vi "GetInputShapeDimCount.vi"(8 "error in (no error)":errorcluster, 10 "inputIndex":i32, 11 "session id in":i32) -> (0 "error out":errorcluster, 2 "InputShapeDimCount":i32, 3 "session id out":i32)   [LabVIEW 2017, in "libonnx_wrapper.lvlib"]
doc: "/**\n * @brief Получить количество размерностей входного тензора\n * \n * Возвращает ранг тензора (число измерений). Например:\n * - Вектор [10] имеет 1 размерность\n * - Матрица [1, 10] имеет 2 размерности\n * - Изображение [1, 3, 224, 224] имеет 4 размерности\n * \n * @param sessionId [IN] ID сессии\n * @param inputIndex [IN] Индекс входа (0-based)\n * \n * @return int32: Количество размерностей (1, 2, 3, 4, ...)\n * @return int32: 0 если сессия не найдена или индекс неверен\n */\nint GetInputShapeDimCount(int sessionId, int inputIndex);"
uses:
  libonnx_wrapper.lvlib
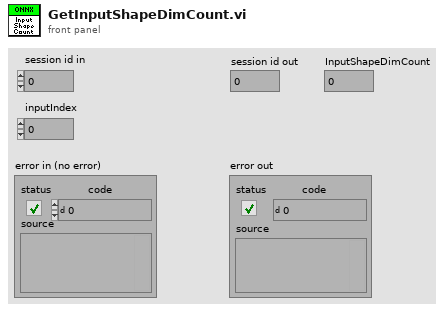
[diagram p1: front panel]
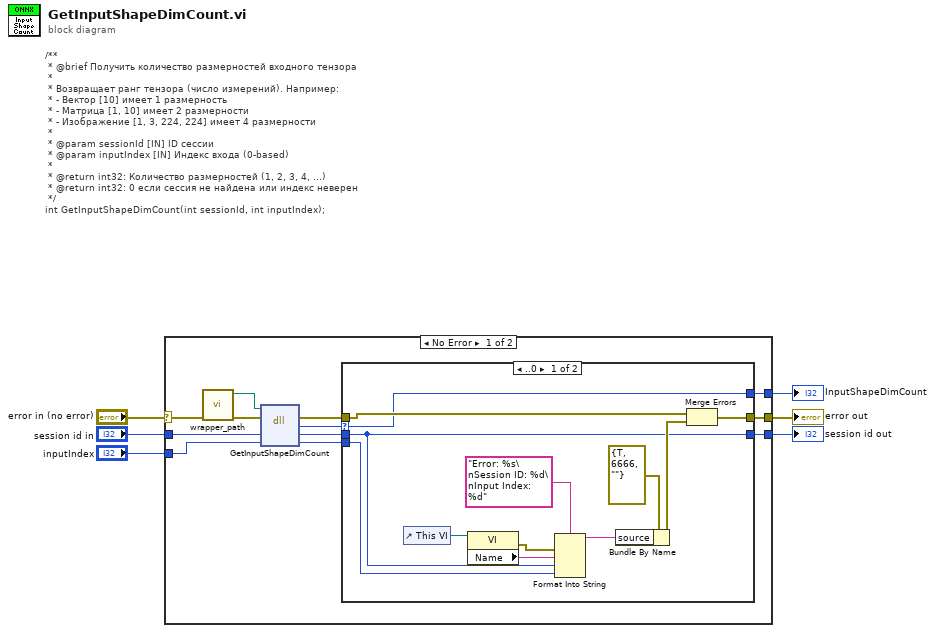
[diagram p0: block diagram]
diagram:
  # "/**\n * @brief Получить количество размерностей входного тензора\n * \n * Возвращает ранг тензора (число измерений). Например:\n * - Вектор [10] имеет 1 размерность\n * - Матрица [1, 10] имеет 2 размерности\n * - Изображение [1, 3, 224, 224] имеет 4 размерности\n * \n * @param sessionId [IN] ID сессии\n * @param inputIndex [IN] Индекс входа (0-based)\n * \n * @return int32: Количество размерностей (1, 2, 3, 4, ...)\n * @return int32: 0 если сессия не найдена или индекс неверен\n */\nint GetInputShapeDimCount(int sessionId, int inputIndex);"
  n1 = case shown="No Error" "error in (no error)" {
    selector: "error in (no error)" -> [w7 w35]
    tunnel: "inputIndex" -> [w18 _]
    tunnel: "session id in" -> [w16 w34]
    tunnel: [w13 w35] -> w4
    tunnel: [w9 _] -> w3
    tunnel: [w8 w34] -> w2
    frame No Error {
      n2 = call "wrapper_path.vi"("error in (no error)"=w7) -> ("error out"=w15:errorcluster, "wrapper path"=w17:path)  [unwired: 9 in]
      n3 = dll-call lib="home/ivan/LabVIEWData/ONNX/Test/libonnx_wrapper/unix64/libonnx_wrapper.so" fn="GetInputShapeDimCount"(path in=w17, error in=w15, "sessionId"=w16, "inputIndex"=w18) -> (error out=w14:errorcluster, "return"=w12:i32, "sessionId"=w11:i32, "inputIndex"=w10:i32)  [unwired: 1 in, 1 out]
      n4 = case shown="..0" w12 {
        selector: w12 -> [w19 w31]
        tunnel: w14 -> [w21 w33]
        tunnel: [w22 w33] -> w13
        tunnel: w11 -> [w23 w32]
        tunnel: [w23 w32] -> w8
        tunnel: w10 -> [w20 _]
        tunnel: [w19 w31] -> w9
        frame ..0 {
          n5 = control-ref of="This VI"() -> (w27:refnum<vi>)
          n6 = property class="VI"(reference=w27) -> (error out=w24:errorcluster, "Name"=w26:string)  [unwired: 1 in, 1 out]
          n7 = Format Into String(format string="Error: %s\nSession ID: %d\nInput Index: %d", error in=w24, w26, w23, w20) -> (resulting string=w28:string)  [unwired: 1 in, 1 out]
          n8 = Bundle By Name(cluster=errorcluster {"status"=TRUE, "code"=6666, "source"=""} ("error out"), "source"=w28) -> (w29:errorcluster)
          n9 = Merge Errors(w21, w29) -> (w22:errorcluster)
        }
        frame 1.. {
        }
      }
    }
    frame Error {
    }
  }
  "error out" <- w4
  "session id out" <- w2
  "InputShapeDimCount" <- w3
